vi "Write RT VI Properties.vi"(8 "Error In":errorcluster, 10 "Supported Targets Properties":T1, 11 "Custom Device .NET Ref In":refnum<k24>) -> (0 "Error Out":errorcluster, 3 "Custom Device .NET Ref Out":refnum<k24>)   [LabVIEW 2015, in "VeriStand XML Parser.lvlib"]
doc: "Sets the properties for each supported target"
uses:
  VeriStand XML Parser.lvlib
  NationalInstruments.VeriStand.XMLReader
  XML Controls/Custom Device Source Distribution Properties.ctl
  XML Controls/Path Cluster.ctl
  XML Controls/Supported Targets.ctl
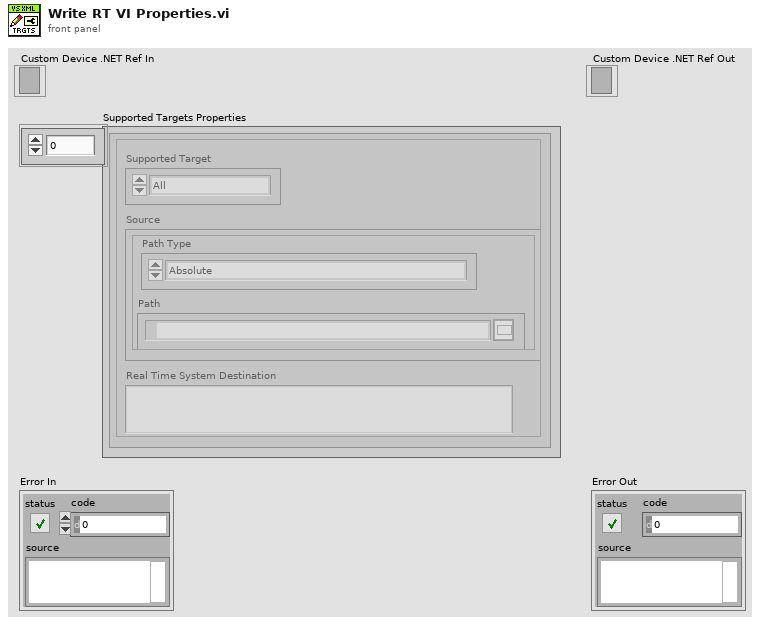
[diagram p1: front panel]
types:
  T1 = typedef "VeriStand XML Parser.lvlib/Custom Device Source Distribution Properties.ctl" = cluster{"Source":T2, "Real Time System Destination":string, "Supported Target":T3}[]
  T2 = typedef "VeriStand XML Parser.lvlib/Path Cluster.ctl" = cluster{"Path":path, "Path Type":enum16{"Absolute", "To Base", "To Common Doc Dir", "To Application Data Dir"}}
  T3 = typedef "VeriStand XML Parser.lvlib/Supported Targets.ctl" = enum16{"All", "Pharlap", "VxWorks", "Windows", "Linux_32_ARM", "Linux_x64", "PharlapWindows", "PharlapVxWorks", "VxWorksWindows"}
  T4 = enum16{"Absolute", "To Base", "To Common Doc Dir", "To Application Data Dir"}
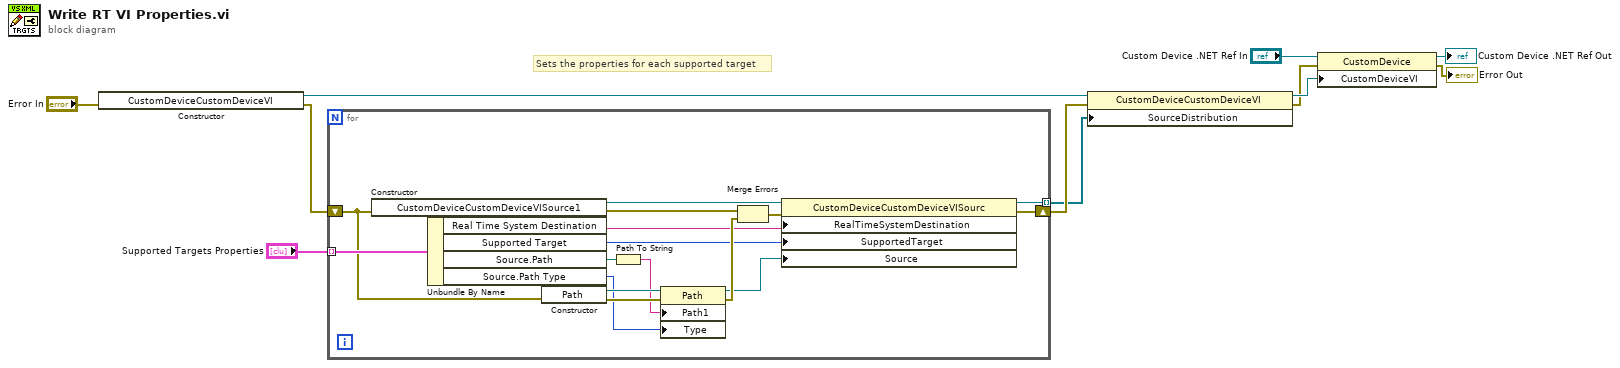
[diagram p0: block diagram]
diagram:
  # "Sets the properties for each supported target"
  n1 = constructor class="CustomDeviceCustomDeviceVI"(error in="Error In") -> (reference out=w5:refnum<k24>, error out=w4:errorcluster)  [unwired: 2 in, 1 out]
  n2 = for {
    shift-right: [w13] -> w7
    shift-left: w4 -> [w23]
    tunnel: "Supported Targets Properties" -> [w27] mode=indexing
    tunnel: [w12] -> w6 mode=indexing
    n3 = constructor class="CustomDeviceCustomDeviceVISourc"(error in=w23) -> (reference out=w26:refnum<k24>, error out=w18:errorcluster)  [unwired: 2 in, 1 out]
    n4 = Unbundle By Name(w27) -> ("Real Time System Destination"=w14:string, "Supported Target"=w15:T3, "Source.Path"=w22:path, "Source.Path Type"=w20:T4)
    n5 = constructor class="Path"(error in=w23) -> (reference out=w25:refnum<k24>, error out=w24:errorcluster)  [unwired: 2 in, 1 out]
    n6 = Path To String(path=w22) -> (string=w21:string)
    n7 = property class="Path"(reference=w25, error in=w24, "Path1"=w21, "Type"=w20) -> (reference out=w16:refnum<k24>, error out=w17:errorcluster)
    n8 = Merge Errors(w18, w17) -> (w19:errorcluster)
    n9 = property class="CustomDeviceCustomDeviceVISourc"(reference=w26, error in=w19, "RealTimeSystemDestination"=w14, "SupportedTarget"=w15, "Source"=w16) -> (reference out=w12:refnum<k24>, error out=w13:errorcluster)
  }
  n10 = property class="CustomDeviceCustomDeviceVI"(reference=w5, error in=w7, "SourceDistribution"=w6) -> (reference out=w9:refnum<k24>, error out=w8:errorcluster)
  n11 = property class="CustomDevice"(reference="Custom Device .NET Ref In", error in=w8, "CustomDeviceVI"=w9) -> (reference out=→"Custom Device .NET Ref Out":refnum<k24>, error out=→"Error Out":errorcluster)
